vi "Toggle Switch.vi"(8 "Button 4":bool, 9 "Button 3":bool, 10 "Button 2":bool, 11 "Button 1":bool) -> (0 "Button 4":bool, 1 "Button 3":bool, 2 "Button 2":bool, 3 "Button 1":bool)   [LabVIEW 2015]
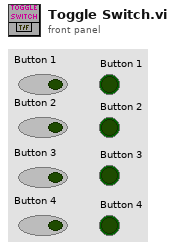
[diagram p1: front panel]
types:
  T1 = cluster{"Button 1":bool, "Button 2":bool, "Button 3":bool, "Button 4":bool}
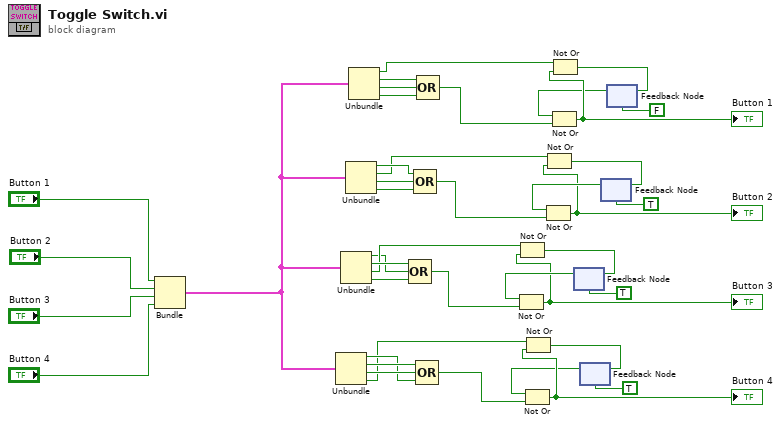
[diagram p0: block diagram]
diagram:
  n1 = Bundle("Button 1"="Button 1", "Button 2"="Button 2", "Button 3"="Button 3", "Button 4"="Button 4") -> (w19:T1)  [unwired: 1 in]
  n2 = Unbundle(w19) -> ("Button 1"=w20:bool, "Button 2"=w22:bool, "Button 3"=w21:bool, "Button 4"=w1:bool)
  n3 = Unbundle(w19) -> ("Button 1"=w23:bool, "Button 2"=w27:bool, "Button 3"=w24:bool, "Button 4"=w26:bool)
  n4 = Unbundle(w19) -> ("Button 1"=w32:bool, "Button 2"=w4:bool, "Button 3"=w34:bool, "Button 4"=w33:bool)
  n5 = Unbundle(w19) -> ("Button 1"=w6:bool, "Button 2"=w37:bool, "Button 3"=w36:bool, "Button 4"=w35:bool)
  n6 = Compound Arithmetic op=OR(w27, w23, w26) -> (w25:bool)
  n7 = Compound Arithmetic op=OR(w32, w34, w33) -> (w3:bool)
  n8 = Compound Arithmetic op=OR(w22, w21, w20) -> (w2:bool)
  n9 = Compound Arithmetic op=OR(w37, w36, w35) -> (w5:bool)
  n10 = feedback #1(TRUE) -> (w31:bool)
  n11 = Not Or(1:w25, 2:w31) -> (0:w29:bool)
  "Button 3" <- w29
  n12 = Not Or(1:w29, 2:w24) -> (0:w30:bool)
  n13 = feedback-in #1(w30) -> ()
  n14 = feedback #2(TRUE) -> (w15:bool)
  n15 = Not Or(1:w2, 2:w15) -> (0:w17:bool)
  "Button 4" <- w17
  n16 = Not Or(1:w17, 2:w1) -> (0:w16:bool)
  n17 = feedback-in #2(w16) -> ()
  n18 = feedback #3(TRUE) -> (w14:bool)
  n19 = Not Or(1:w3, 2:w14) -> (0:w12:bool)
  "Button 2" <- w12
  n20 = Not Or(1:w12, 2:w4) -> (0:w13:bool)
  n21 = feedback-in #3(w13) -> ()
  n22 = feedback #4(FALSE) -> (w7:bool)
  n23 = Not Or(1:w5, 2:w7) -> (0:w9:bool)
  "Button 1" <- w9
  n24 = Not Or(1:w9, 2:w6) -> (0:w8:bool)
  n25 = feedback-in #4(w8) -> ()
